vi "Globals.vi"() -> ()   [LabVIEW 2025]
uses:
  State.ctl
  Mode.ctl
panel:
  in  "PicoCfgChng":bool
  out "Tn":timestamp
  out "Wh":dbl
  out "Ah":dbl
  in  "I":dbl[](array[numeric])
  in  "V":dbl[](array[numeric])
  in  "T":dbl[](array[numeric])
  out "FileRefnum":refnum<file>
  out "LastFile":path
  out "T0":timestamp
  out "R":dbl[](array[numeric])=[0.19948381185531616, 0.39327406883239746, 0.3932740092277527]
  out "CalStart":timestamp
  in  "Mode":T1=enum."Serial"
  in  "State":T2
  in  "Calibration":sgl[](array[numeric])
  out "ConnPort":refnum<visa-resource-name>
  # "R1 Only"
  # "Serial"
  # "Parallel"
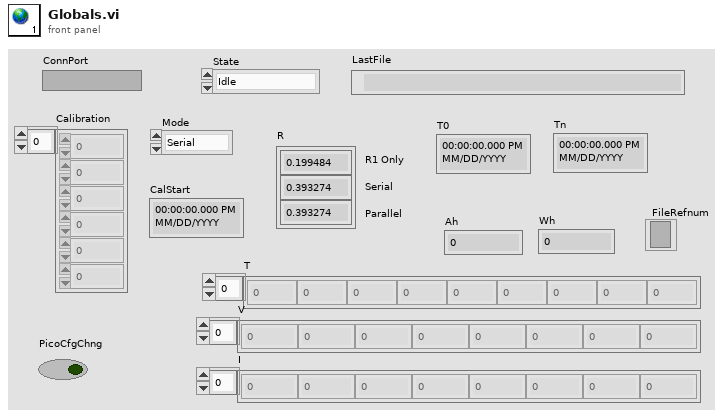
[diagram p1: front panel]
types:
  T1 = typedef "Mode.ctl" = enum16{"R1 Only", "Parallel", "Serial"}
  T2 = typedef "State.ctl" = enum16{"Idle", "Connected", "Calibrating", "Running", "Sync"}
diagram:
